vi "Autonomous Independent.vi"   [LabVIEW 2015]
doc: "This VI is called when autonomous begins, and will automatically be terminated when autonomous ends. You can carry out timed or sensor driven robot movement independently without needing to return to the caller."
uses:
  Robot Global Data.vi
panel:
  # "AUTONOMOUS INDEPENDENT.VI"
  # "Drive Modes:\n     ( 0) - Driver Control\n     ( 1) - Constant Velocity, Turn Right, Slow\n     ( 2) - Constant Velocity, Turn Left, Slow\n     ( 3) - Constant Velocity, Go Straight, Slow"
types:
  T1 = typedef "WPI_MotorControlDeviceRef.ctl" = cluster{"DeviceStatus":errorcluster, "Type":T2, "PWM":cluster{"PWM Channel":T3, "DeadBand":T4}, "CAN":cluster{"Device Number":u8, "Control Mode":T5, "Semaphore":T6, "Max Vout":dbl, "TalonSRX Control Mode":T7}, "Invert":bool}
  T2 = typedef "WPI_MotorControlType.ctl" = enum16{"PWM", "CAN", "CANTalonSRX"}
  T3 = typedef "FPGA_DIOPWMChannel.ctl" = enum8{"PWM 0", "PWM 1", "PWM 2", "PWM 3", "PWM 4", "PWM 5", "PWM 6", "PWM 7", "PWM 8", "PWM 9", "PWM MXP 0", "PWM MXP 1", "PWM MXP 2", "PWM MXP 3", "PWM MXP 4", "PWM MXP 5", "PWM MXP 6", "PWM MXP 7", "PWM MXP 8", "PWM MXP 9", "Invalid"}
  T4 = typedef "WPI_PWMDeadband.ctl" = cluster{"Name":string, "maxPositivePwm":i32, "minPositivePwm":i32, "centerPwm":i32, "maxNegativePwm":i32, "minNegativePwm":i32, "angularRange":u16}
  T5 = typedef "WPI_CANJaguar_ControlMode.ctl" = enum8{"Percent VBus", "Current", "Speed", "Position", "Voltage"}
  T6 = typedef "Semaphore RefNum" = refnum<k1>
  T7 = typedef "WPI_CANTalonSRX_APIControlMode.ctl" = enum8{"Percent VBus", "Speed", "Position", "Slave", "Unchanged / Invalid", "Voltage Compensation", "Current", "Motion Profile"}
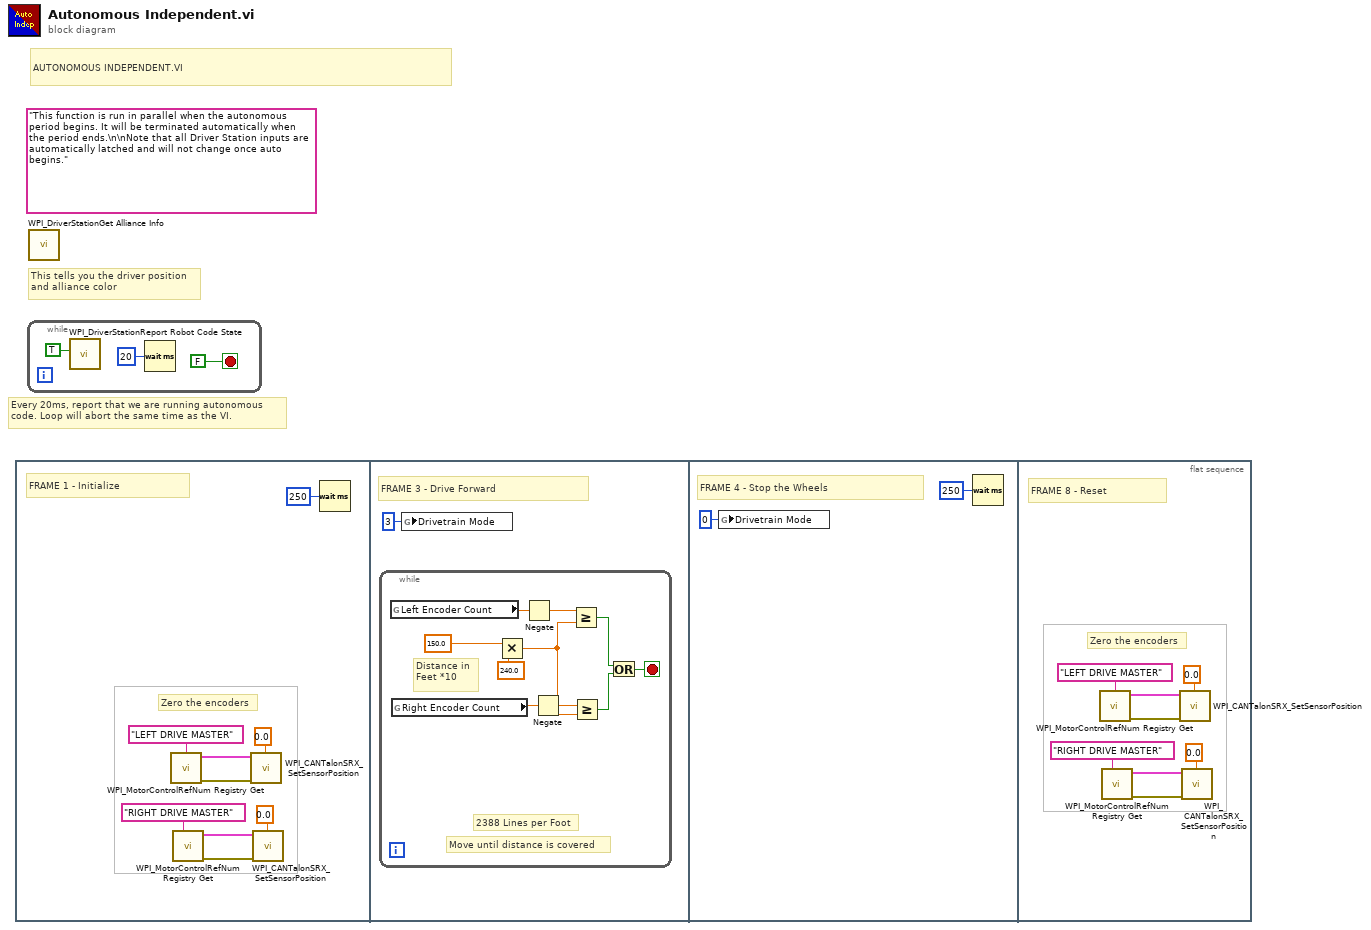
[diagram p0: block diagram]
diagram:
  (unwired) "This function is run in parallel when the autonomous period begins. It will be terminated automatically when the period ends.\n\nNote that all Driver Station inputs are automatically latched and will not change once auto begins."
  # "AUTONOMOUS INDEPENDENT.VI"
  # "Every 20ms, report that we are running autonomous\ncode. Loop will abort the same time as the VI."
  # "This tells you the driver position\nand alliance color"
  n1 = flat-sequence {
    frame #0 {
      # "Zero the encoders"
      # "FRAME 1 - Initialize"
      n2 = call <vilib>:"WPI_MotorControlRefNum Registry Get.vi"("refnum name"="LEFT DRIVE MASTER") -> ("error out"=w8:errorcluster, "MotorControlDevRef"=w7:T1)  [unwired: 9 in]
      n3 = call <vilib>:"WPI_MotorControlRefNum Registry Get.vi"("refnum name"="RIGHT DRIVE MASTER") -> ("error out"=w4:errorcluster, "MotorControlDevRef"=w3:T1)  [unwired: 9 in]
      n4 = call <vilib>:"WPI_CANTalonSRX_SetSensorPosition.vi"("error in (no error)"=w8, "New Sensor Position"=0.0, "CAN Talon SRX Ref"=w7) -> ()  [unwired: 7 in, 2 out]
      n5 = call <vilib>:"WPI_CANTalonSRX_SetSensorPosition.vi"("error in (no error)"=w4, "New Sensor Position"=0.0, "CAN Talon SRX Ref"=w3) -> ()  [unwired: 7 in, 2 out]
      n6 = Wait (ms)(milliseconds to wait=u32 250) -> ()  [unwired: 1 out]
    }
    frame #1 {
      # "FRAME 3 - Drive Forward"
      n7 = while {
        stop <- w18 stop-if-true
        # "Distance in Feet *10"
        # "Move until distance is covered"
        # "2388 Lines per Foot"
        n8 = global read "Robot Global Data.vi" "Left Encoder Count"() -> (w14:dbl)
        n9 = global read "Robot Global Data.vi" "Right Encoder Count"() -> (w11:dbl)
        n10 = Multiply(x=150.0 ("y"), y=240.0) -> (x*y=w15:dbl)
        n11 = Negate(x=w14) -> (-x=w13:dbl)
        n12 = Negate(x=w11) -> (-x=w12:dbl)
        n13 = Greater Or Equal?(x=w13, y=w15) -> (x >= y?=w20:bool)
        n14 = Greater Or Equal?(x=w12, y=w15) -> (x >= y?=w19:bool)
        n15 = Or(x=w20, y=w19) -> (x .or. y?=w18:bool)
      }
      n16 = global write "Robot Global Data.vi" "Drivetrain Mode"(u16 3 ("Ball Lift Lowered Target")) -> ()
    }
    frame #2 {
      # "FRAME 4 - Stop the Wheels"
      n17 = global write "Robot Global Data.vi" "Drivetrain Mode"(u16 0 ("Ball Lift Lowered Target")) -> ()
      n18 = Wait (ms)(milliseconds to wait=u32 250) -> ()  [unwired: 1 out]
    }
    frame #3 {
      # "Zero the encoders"
      # "FRAME 8 - Reset"
      n19 = call <vilib>:"WPI_MotorControlRefNum Registry Get.vi"("refnum name"="LEFT DRIVE MASTER") -> ("error out"=w29:errorcluster, "MotorControlDevRef"=w28:T1)  [unwired: 9 in]
      n20 = call <vilib>:"WPI_MotorControlRefNum Registry Get.vi"("refnum name"="RIGHT DRIVE MASTER") -> ("error out"=w25:errorcluster, "MotorControlDevRef"=w24:T1)  [unwired: 9 in]
      n21 = call <vilib>:"WPI_CANTalonSRX_SetSensorPosition.vi"("error in (no error)"=w29, "New Sensor Position"=0.0, "CAN Talon SRX Ref"=w28) -> ()  [unwired: 7 in, 2 out]
      n22 = call <vilib>:"WPI_CANTalonSRX_SetSensorPosition.vi"("error in (no error)"=w25, "New Sensor Position"=0.0, "CAN Talon SRX Ref"=w24) -> ()  [unwired: 7 in, 2 out]
    }
  }
  n23 = while {
    stop <- FALSE stop-if-true
    n24 = call <vilib>:"WPI_DriverStationReport Robot Code State.vi"("Autonomous"=TRUE) -> ()  [unwired: 10 in, 1 out]
    n25 = Wait (ms)(milliseconds to wait=u32 20) -> ()  [unwired: 1 out]
  }
  n26 = call <vilib>:"WPI_DriverStationGet Alliance Info.vi"() -> ()  [unwired: 12 out]
